vi "Configure Crop.vi"(6 "Codec":string, 8 "error in (no error)":errorcluster, 9 "Time Crop Method":T1, 11 "Frame Grabber Data In":T2={"Camera Session"="", "Frame"=refnum, "AVI Refnum"=refnum, "Codecs"=[], "Frame number"=0, "Tracking File Refnum"=refnum, "Tick Count"=0, "Probe Object"=refnum, "Playback Probe Data"=[], "Rigid Body"={"Position"={"x (mm)"=0.0, "y (mm)"=0.0, "z (mm)"=0.0}, "Orientation"={"Pitch (rad)"=0.0, "Yaw (rad)"=0.0, "Roll (rad)"=0.0}, "Quaternion"={"qx"=0.0, "qy"=0.0, "qz"=0.0, "qw"=0.0}, "Tracked?"=FALSE}, "Total no frames playback"=0, "Video FPS"=0.0, "Camera connected?"=FALSE, "Scene"=refnum, "Cropped Frame"=refnum, "Tracker FPS"=0.0, "Crop ROI"=[], "Presentation Values"=[], "Elapsed time (ms)"=0, "Camera frames playback"=0, "Refnums"={"Live Refnum"=refnum, "Record Refnum"=refnum, "Playback Refnum"=refnum, "Frame Slider Refnum"=refnum, "Pause Refnum"=refnum, "Home Refnum"=refnum, "Crop Refnum"=refnum, "Clear Crop Refnum"=refnum, "stop refnum"=refnum, "Playback Rate Refnum"=refnum, "Presentation Refnum"=refnum, "Crop Time Frame Slider Refnum"=refnum, "Cancel Save Refnum"=refnum, "Reverse Playback Refnum"=refnum, "Recording Settings Refnum"=refnum, "Camera Frame Refnum"=refnum}, "Dimensions"={"Probe Dimensions"={"Probe Width"=0.0, "Probe Depth"=1.0, "Probe Height"=0.0}, "Room Dimensions"={"Room Width"=0.0, "Room Depth"=0.0, "Room Height"=0.0}}, "Playback Data As Strings"=[], "Cropped Tracking File Refnum"=refnum, "Cropped AVI Refnum"=refnum, "Header"=[], "Total euclidian distance"=0.0, "Annotation File Path"=path "", "Playback File Path"=path "", "Size per frame"=0.0}) -> (0 "error out":errorcluster, 1 "Valid crop region?":bool, 2 "Saving?":bool, 3 "Frame Grabber Data Out":T2={"Camera Session"="", "Frame"=refnum, "AVI Refnum"=refnum, "Codecs"=[], "Frame number"=0, "Tracking File Refnum"=refnum, "Tick Count"=0, "Probe Object"=refnum, "Playback Probe Data"=[], "Rigid Body"={"Position"={"x (mm)"=0.0, "y (mm)"=0.0, "z (mm)"=0.0}, "Orientation"={"Pitch (rad)"=0.0, "Yaw (rad)"=0.0, "Roll (rad)"=0.0}, "Quaternion"={"qx"=0.0, "qy"=0.0, "qz"=0.0, "qw"=0.0}, "Tracked?"=FALSE}, "Total no frames playback"=0, "Video FPS"=0.0, "Camera connected?"=FALSE, "Scene"=refnum, "Cropped Frame"=refnum, "Tracker FPS"=0.0, "Crop ROI"=[], "Presentation Values"=[], "Elapsed time (ms)"=0, "Camera frames playback"=0, "Refnums"={"Live Refnum"=refnum, "Record Refnum"=refnum, "Playback Refnum"=refnum, "Frame Slider Refnum"=refnum, "Pause Refnum"=refnum, "Home Refnum"=refnum, "Crop Refnum"=refnum, "Clear Crop Refnum"=refnum, "stop refnum"=refnum, "Playback Rate Refnum"=refnum, "Presentation Refnum"=refnum, "Crop Time Frame Slider Refnum"=refnum, "Cancel Save Refnum"=refnum, "Reverse Playback Refnum"=refnum, "Recording Settings Refnum"=refnum, "Camera Frame Refnum"=refnum}, "Dimensions"={"Probe Dimensions"={"Probe Width"=0.0, "Probe Depth"=1.0, "Probe Height"=0.0}, "Room Dimensions"={"Room Width"=0.0, "Room Depth"=0.0, "Room Height"=0.0}}, "Playback Data As Strings"=[], "Cropped Tracking File Refnum"=refnum, "Cropped AVI Refnum"=refnum, "Header"=[], "Total euclidian distance"=0.0, "Annotation File Path"=path "", "Playback File Path"=path "", "Size per frame"=0.0})   [LabVIEW 2017]
uses:
  Controls/Frame Grabber Data.ctl
  <vilib>/userdefined/High Color/IMAQdx.ctl
  <vilib>/vision/Image Controls.llb/IMAQ Image.ctl
  <vilib>/vision/Avi.llb/IMAQ AVI2 Refnum.ctl
  Controls/Rigid Body Info.ctl
  Controls/Position.ctl
  Controls/Orientation.ctl
  Controls/Refnums.ctl
  Controls/Recording Settings.ctl
  Controls/Operator Settings.ctl
  Controls/Operator.ctl
  Controls/Patient Settings.ctl
  Controls/Dimensions.ctl
  Controls/Room Dimensions.ctl
  Controls/Time Crop Method.ctl
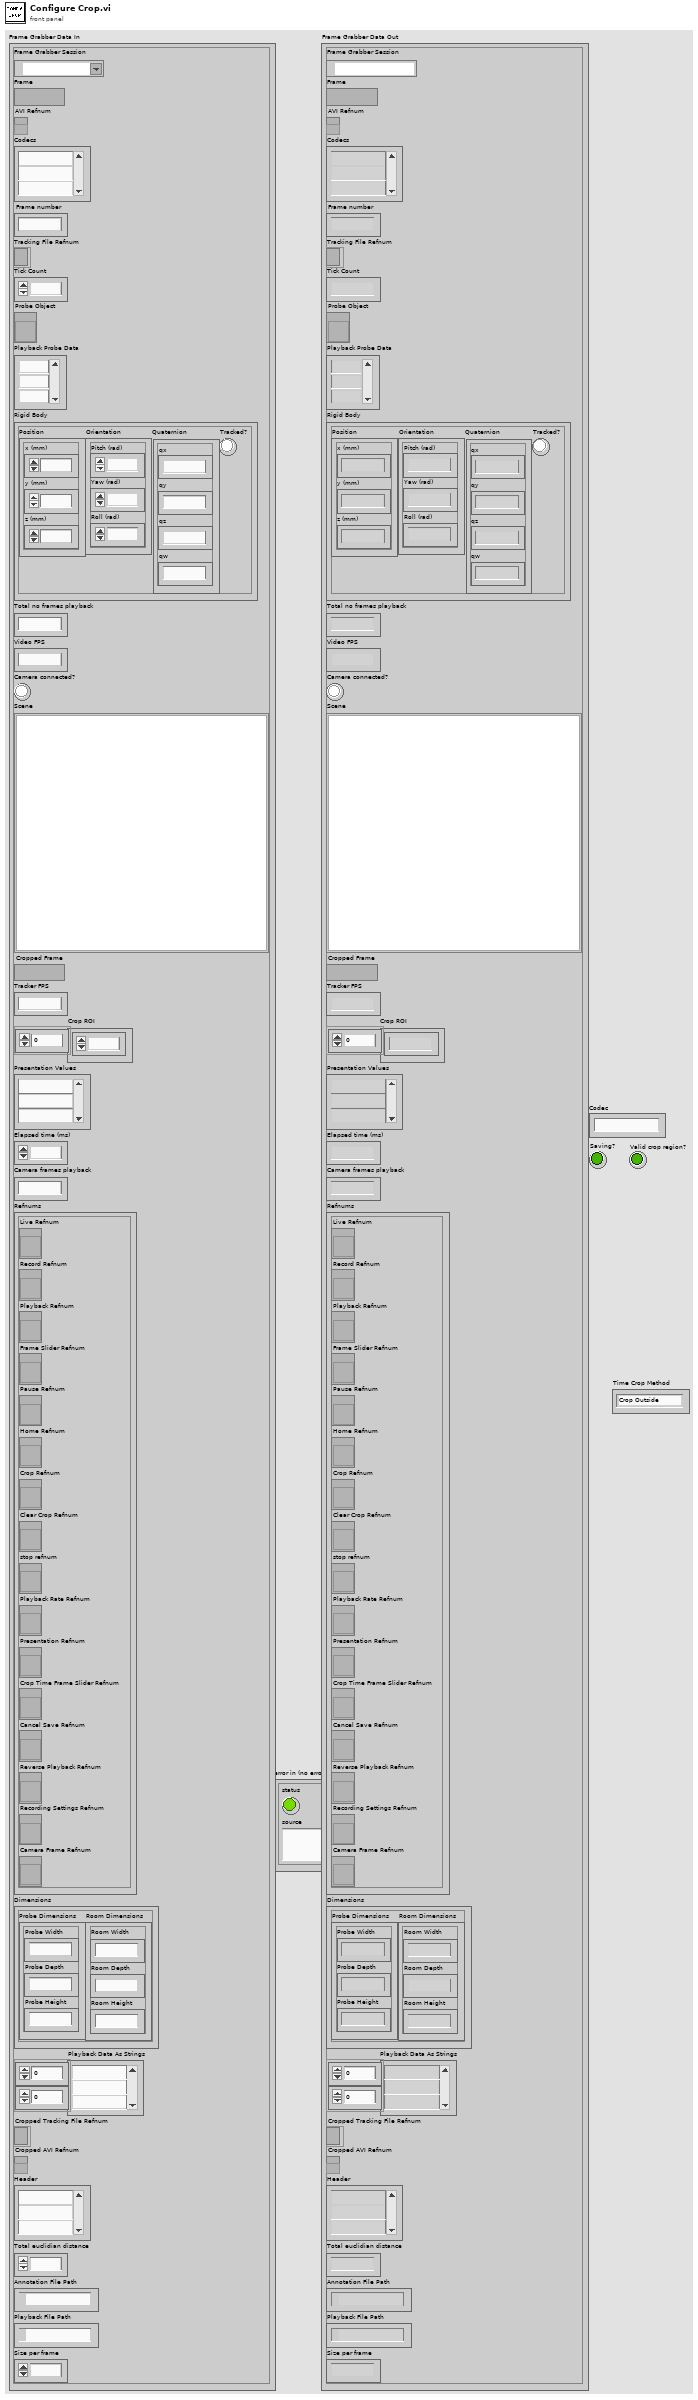
[diagram p1: front panel]
types:
  T1 = typedef "Time Crop Method.ctl" = enum16{"Crop Outside", "Crop Inside"}
  T2 = typedef "Frame Grabber Data.ctl" = cluster{"Camera Session":T3, "Frame":T4, "AVI Refnum":T5, "Codecs":string[], "Frame number":u32, "Tracking File Refnum":refnum<file>, "Tick Count":u32, "Probe Object":refnum<vi>, "Playback Probe Data":dbl[][], "Rigid Body":T6, "Total no frames playback":i32, "Video FPS":dbl, "Camera connected?":bool, "Scene":refnum<vi>, "Cropped Frame":T4, "Tracker FPS":dbl, "Crop ROI":i32[], "Presentation Values":string[], "Elapsed time (ms)":u32, "Camera frames playback":u32, "Refnums":T9, "Dimensions":T10, "Playback Data As Strings":string[][], "Cropped Tracking File Refnum":refnum<file>, "Cropped AVI Refnum":T5, "Header":string[], "Total euclidian distance":dbl, "Annotation File Path":path, "Playback File Path":path, "Size per frame":dbl}
  T3 = typedef "IMAQdx.ctl" = refnum<k21>
  T4 = typedef "IMAQ Image.ctl" = refnum<image>
  T5 = typedef "IMAQ AVI2 Refnum.ctl" = refnum<k20>
  T6 = typedef "Rigid Body Info.ctl" = cluster{"Position":T7, "Orientation":T8, "Quaternion":cluster{"qx":sgl, "qy":sgl, "qz":sgl, "qw":sgl}, "Tracked?":bool}
  T7 = typedef "Position.ctl" = cluster{"x (mm)":sgl, "y (mm)":sgl, "z (mm)":sgl}
  T8 = typedef "Orientation.ctl" = cluster{"Pitch (rad)":sgl, "Yaw (rad)":sgl, "Roll (rad)":sgl}
  T9 = typedef "Refnums.ctl" = cluster{"Live Refnum":refnum<vi>, "Record Refnum":refnum<vi>, "Playback Refnum":refnum<vi>, "Frame Slider Refnum":refnum<vi>, "Pause Refnum":refnum<vi>, "Home Refnum":refnum<vi>, "Crop Refnum":refnum<vi>, "Clear Crop Refnum":refnum<vi>, "stop refnum":refnum<vi>, "Playback Rate Refnum":refnum<vi>, "Presentation Refnum":refnum<vi>, "Crop Time Frame Slider Refnum":refnum<vi>, "Cancel Save Refnum":refnum<vi>, "Reverse Playback Refnum":refnum<vi>, "Recording Settings Refnum":refnum<vi>, "Camera Frame Refnum":refnum<vi>}
  T10 = typedef "Dimensions.ctl" = cluster{"Probe Dimensions":cluster{"Probe Width":sgl, "Probe Depth":sgl, "Probe Height":sgl}, "Room Dimensions":T11}
  T11 = typedef "Room Dimensions.ctl" = cluster{"Room Width":dbl, "Room Depth":dbl, "Room Height":dbl}
  T12 = enum16{"open", "replace", "create", "open or create", "replace or create", "replace or create with confirmation"}
  T13 = cluster{"Width":u32, "Height":u32, "Frames Per Second":u32, "Codec":string, "Has Data":bool}
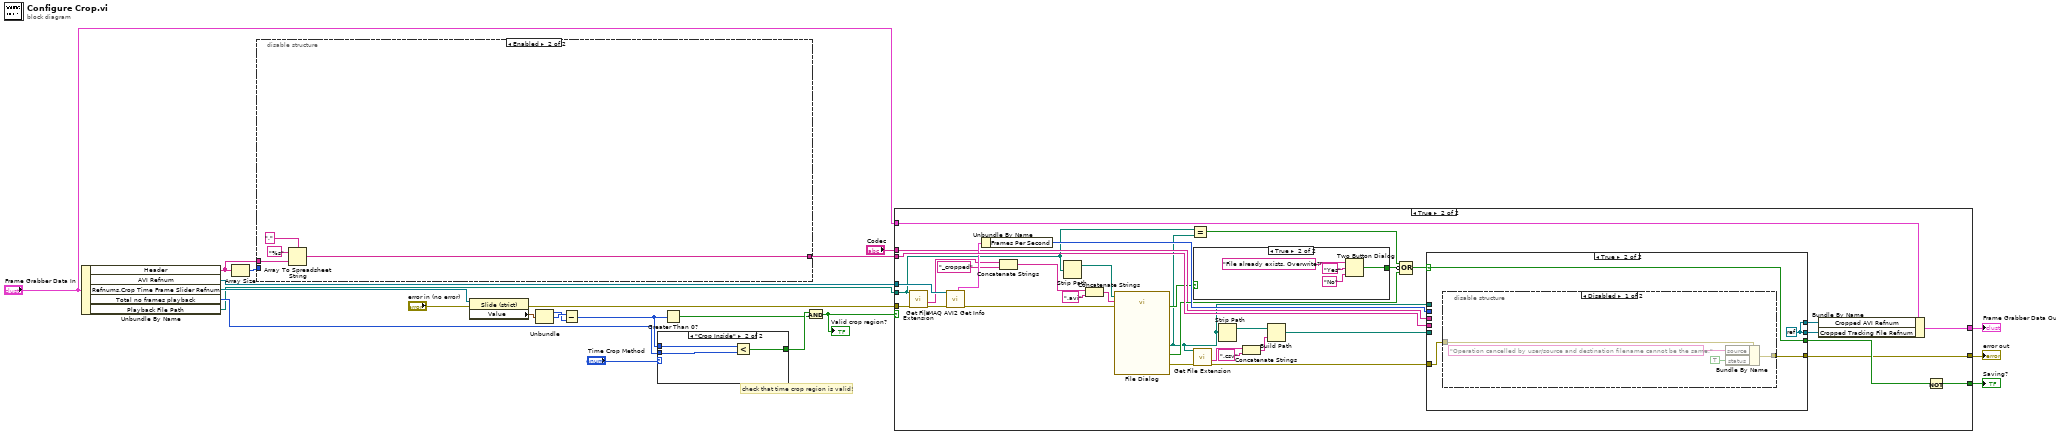
[diagram p0: block diagram]
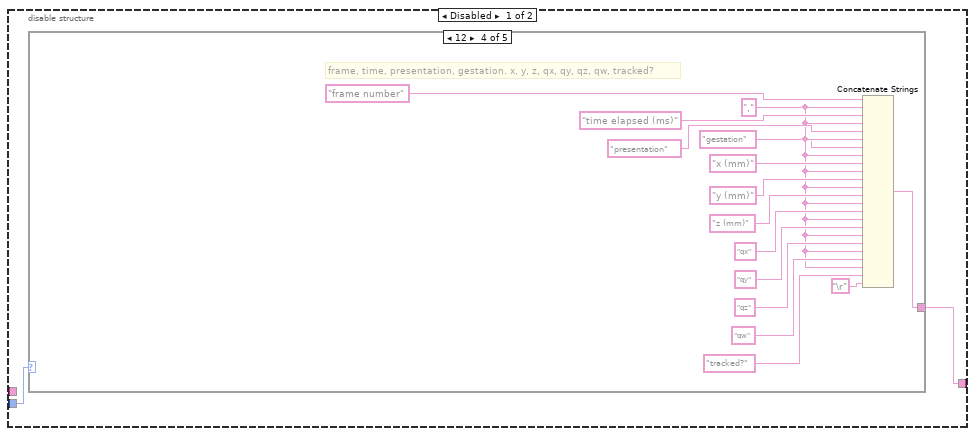
[diagram p2: hidden frame]
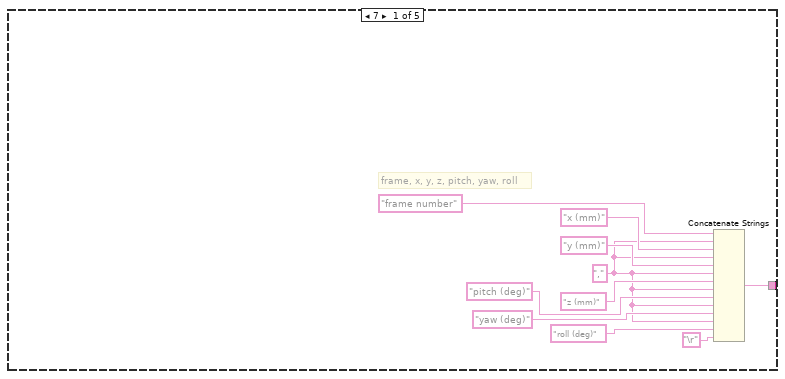
[diagram p3: hidden frame]
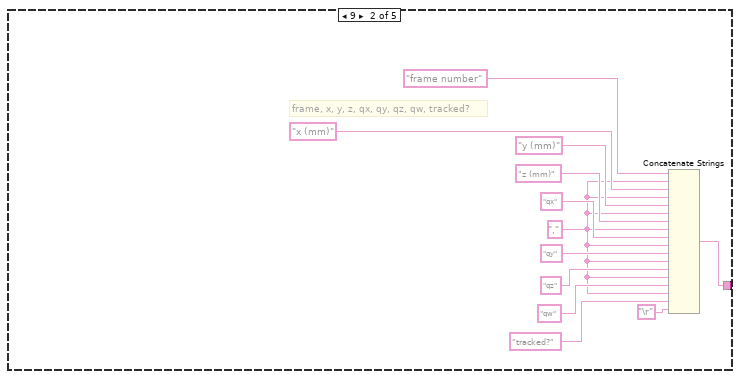
[diagram p4: hidden frame]
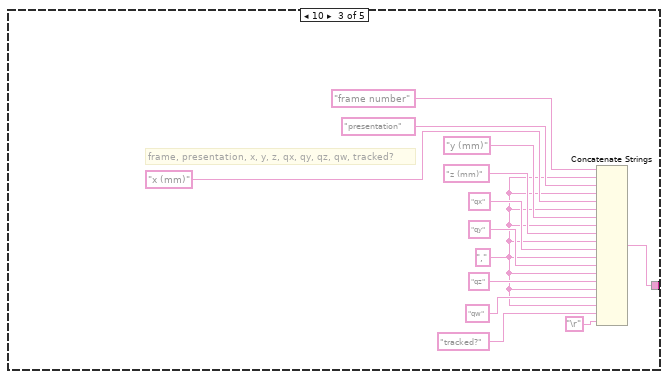
[diagram p5: hidden frame]
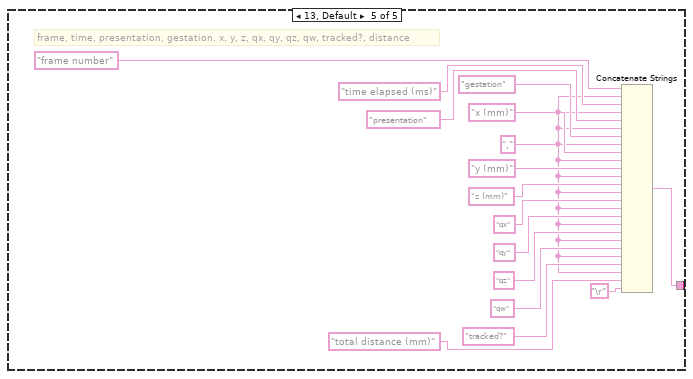
[diagram p6: hidden frame]
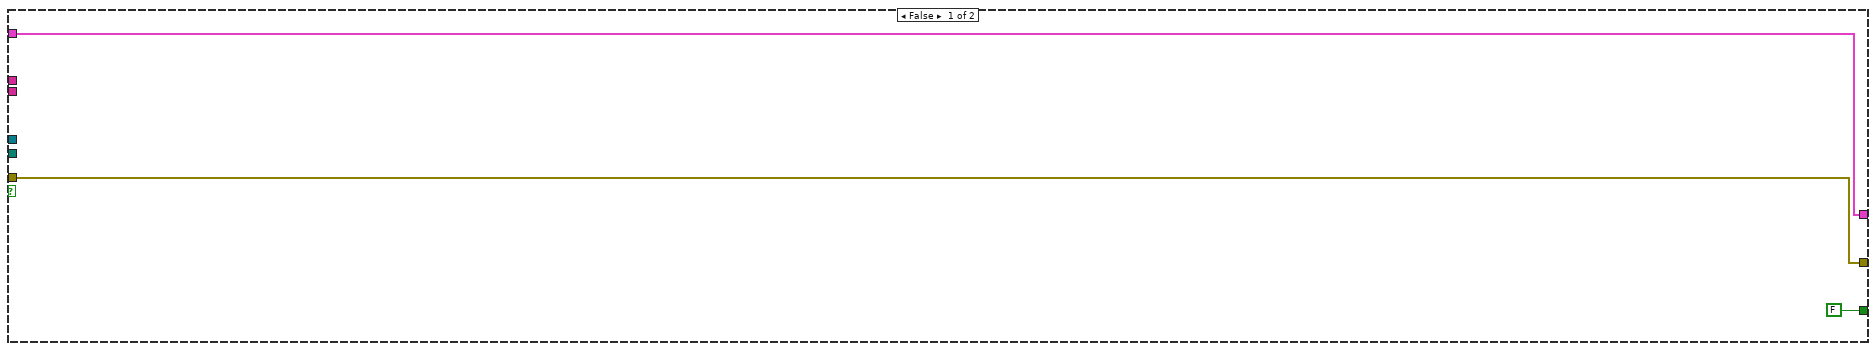
[diagram p7: hidden frame]
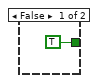
[diagram p8: hidden frame]
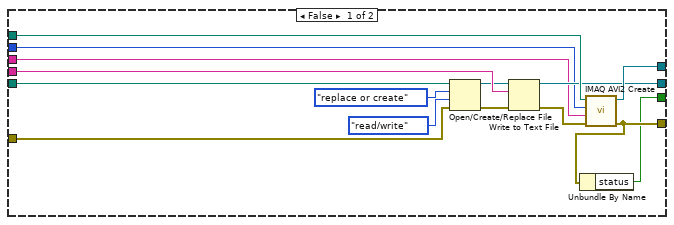
[diagram p9: hidden frame]
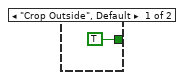
[diagram p11: hidden frame]
diagram:
  # "check that time crop region is valid!"
  n1 = Unbundle By Name("Frame Grabber Data In") -> ("Header"=w1:string[], "AVI Refnum"=w19:T5, "Refnums.Crop Time Frame Slider Refnum"=w15:refnum<vi>, "Total no frames playback"=w12:i32, "Playback File Path"=w4:path)
  n2 = Array Size(array=w1) -> (size(s)=w3:i32)
  n3 = disable-structure shown="Enabled" {
    disable-tunnel: [w24 w91] -> w22
    disable-tunnel: w3 -> [w23 _]
    disable-tunnel: w1 -> [_ w93]
    frame Disabled {
      n4 = case shown="12" w23 {
        tunnel: [w26 w37 w47 w74 w90] -> w24
        frame 7 {
          w25 = ","
          # "frame, x, y, z, pitch, yaw, roll"
          n5 = Concatenate Strings("frame number" ("string"), w25, "x (mm)" ("string"), w25, "y (mm)" ("string"), w25, "z (mm)" ("string"), w25, "pitch (deg)" ("string"), w25, "yaw (deg)" ("string"), w25, "roll (deg)" ("string"), "\r") -> (w26:string)
        }
        frame 9 {
          w38 = ","
          # "frame, x, y, z, qx, qy, qz, qw, tracked?"
          n6 = Concatenate Strings("frame number" ("string"), w38, "x (mm)" ("string"), w38, "y (mm)" ("string"), w38, "z (mm)" ("string"), w38, "qx" ("string"), w38, "qy" ("string"), w38, "qz" ("string"), w38, "qw" ("string"), w38, "tracked?" ("string"), "\r") -> (w37:string)
        }
        frame 10 {
          w49 = ","
          # "frame, presentation, x, y, z, qx, qy, qz, qw, tracked?"
          n7 = Concatenate Strings("frame number" ("string"), w49, "presentation" ("string"), w49, "x (mm)" ("string"), w49, "y (mm)" ("string"), w49, "z (mm)" ("string"), w49, "qx" ("string"), w49, "qy" ("string"), w49, "qz" ("string"), w49, "qw" ("string"), w49, "tracked?" ("string"), "\r") -> (w47:string)
        }
        frame 12 {
          w61 = ","
          # "frame, time, presentation, gestation. x, y, z, qx, qy, qz, qw, tracked?"
          n8 = Concatenate Strings("frame number" ("string"), w61, "time elapsed (ms)" ("string"), w61, "presentation" ("string"), w61, "gestation" ("string"), w61, "x (mm)" ("string"), w61, "y (mm)" ("string"), w61, "z (mm)" ("string"), w61, "qx" ("string"), w61, "qy" ("string"), w61, "qz" ("string"), w61, "qw" ("string"), w61, "tracked?" ("string"), "\r") -> (w74:string)
        }
        frame 13, Default {
          w76 = ","
          # "frame, time, presentation, gestation. x, y, z, qx, qy, qz, qw, tracked?, distance"
          n9 = Concatenate Strings("frame number" ("string"), w76, "time elapsed (ms)" ("string"), w76, "presentation" ("string"), w76, "gestation" ("string"), w76, "x (mm)" ("string"), w76, "y (mm)" ("string"), w76, "z (mm)" ("string"), w76, "qx" ("string"), w76, "qy" ("string"), w76, "qz" ("string"), w76, "qw" ("string"), w76, "tracked?" ("string"), w76, "total distance (mm)" ("string"), "\r") -> (w90:string)
        }
      }
    }
    frame Enabled {
      n10 = Array To Spreadsheet String(delimiter (Tab)=",", array=w93, 3:"%s" ("format string")) -> (spreadsheet string=w91:string)
    }
  }
  n11 = property class="Slide (strict)"(reference=w15, error in="error in (no error)") -> (error out=w9:errorcluster, "Value"=w16:cluster{i32, i32, i32})  [unwired: 1 out]
  n12 = Unbundle(w16) -> (w17:i32, w18:i32)  [unwired: 1 out]
  n13 = Subtract(x=w18, y=w17) -> (x-y=w13:i32)
  n14 = case shown="\"Crop Inside\"" "Time Crop Method" {
    tunnel: w13 -> [_ w97]
    tunnel: w12 -> [_ w96]
    tunnel: [TRUE w98] -> w11
    frame "Crop Outside", Default {
    }
    frame "Crop Inside" {
      n15 = Less?(x=w97, y=w96) -> (x < y?=w98:bool)
    }
  }
  n16 = Greater Than 0?(x=w13) -> (x > 0?=w8:bool)
  n17 = And(x=w11, y=w8) -> (x .and. y?=w6:bool)
  "Valid crop region?" <- w6
  n18 = case shown="True" w6 {
    tunnel: w22 -> [_ w136]
    tunnel: "Frame Grabber Data In" -> [w100 w135]
    tunnel: [w100 w130] -> w20
    tunnel: w19 -> [_ w128]
    tunnel: w9 -> [w99 w121]
    tunnel: w4 -> [_ w110]
    tunnel: [FALSE ("status") w120] -> w7
    tunnel: "Codec" -> [_ w115]
    tunnel: [w99 w102] -> w2
    frame False {
    }
    frame True {
      n19 = call <vilib>:"Get File Extension.vi"("error in (no error)"=w121, "file"=w110) -> ("error out"=w123:errorcluster, "filename without extension"=w125:string)  [unwired: 5 in, 3 out]
      n20 = call "IMAQ AVI2 Get Info"("error in (no error)"=w123, "AVI Refnum"=w128) -> ("error out"=w119:errorcluster, "Frame Data"=w127:T13)  [unwired: 5 in, 3 out]
      n21 = Unbundle By Name(w127) -> ("Frames Per Second"=w126:u32)
      n22 = Concatenate Strings(w125, "_cropped" ("string")) -> (w122:string)
      n23 = Strip Path(path=w110) -> (stripped path=w114:path)  [unwired: 1 out]
      n24 = Concatenate Strings(w122, ".avi" ("string")) -> (w118:string)
      n25 = call "File Dialog"("start path"=w114, "default name"=w118, "error in"=w119) -> ("selected path"=w109:path, "exists"=w111:bool, "cancelled"=w116:bool, "error out"=w112:errorcluster)  [unwired: 9 in]
      n26 = Equal?(x=w110, y=w109) -> (x = y?=w107:bool)
      n27 = case shown="True" w111 {
        tunnel: [TRUE ("T button?") w140] -> w106
        frame False {
        }
        frame True {
          n28 = Two Button Dialog(message="File already exists. Overwrite?", 1:"No" ("F button name (\"Cancel\")"), 2:"Yes" ("T button name (\"OK\")")) -> (T button?=w140:bool)
        }
      }
      n29 = call <vilib>:"Get File Extension.vi"("error in (no error)"=w112, "file"=w109) -> ("error out"=w105:errorcluster, "filename without extension"=w113:string)  [unwired: 5 in, 3 out]
      n30 = Strip Path(path=w109) -> (stripped path=w108:path)  [unwired: 1 out]
      n31 = Concatenate Strings(w113, ".csv" ("string")) -> (w133:string)
      n32 = Build Path(base path=w108, name or relative path=w133) -> (appended path=w104:path)
      n33 = Compound Arithmetic op=OR(w107, invert w106, w116) -> (w117:bool)
      n34 = case shown="True" w117 {
        selector: w117 -> [_ w157]
        tunnel: w136 -> [w156 _]
        tunnel: [w155 w160] -> w131
        tunnel: w109 -> [w154 _]
        tunnel: [w153 w160] -> w129
        tunnel: w115 -> [w152 _]
        tunnel: w126 -> [w151 _]
        tunnel: [w149 w159] -> w102
        tunnel: w105 -> [w148 w158]
        tunnel: w104 -> [w145 _]
        tunnel: [w142 w157] -> w103
        frame False {
          n35 = Open/Create/Replace File(file path (use dialog)=w145, error in=w148, operation (0:open)=T12."replace or create", access (0:read/write)=enum16{"read/write", "read-only", "write-only"}."read/write") -> (refnum out=w143:refnum<file>, error out=w144:errorcluster)  [unwired: 2 in, 1 out]
          n36 = Write to Text File(file (use dialog)=w143, text=w156, error in=w144) -> (refnum out=w153:refnum<file>, error out=w150:errorcluster)  [unwired: 1 in, 1 out]
          n37 = call "IMAQ AVI2 Create"("error in (no error)"=w150, "Codec"=w152, "Frames Per Second"=w151, "AVI Path"=w154) -> ("error out"=w149:errorcluster, "AVI Refnum"=w155:T5)  [unwired: 6 in]
          n38 = Unbundle By Name(w149) -> ("status"=w142:bool)
        }
        frame True {
          w160 = refnum<k0> refnum
          n39 = disable-structure shown="Disabled" {
            disable-tunnel: [w164 w165] -> w159
            disable-tunnel: w158 -> [w161 w165]
            frame Disabled {
              n40 = Bundle By Name(cluster=w161, "source"="Operation cancelled by user/source and destination filename cannot be the same.", "status"=TRUE) -> (w164:errorcluster)
            }
            frame Enabled {
            }
          }
        }
      }
      n41 = Bundle By Name(cluster=w135, "Cropped AVI Refnum"=w131, "Cropped Tracking File Refnum"=w129) -> (w130:T2)
      n42 = Not(x=w103) -> (.not. x?=w120:bool)
    }
  }
  "Frame Grabber Data Out" <- w20
  "Saving?" <- w7
  "error out" <- w2
